vi "Puzzle 16-2 right.vi"() -> ()   [LabVIEW 2022 SP3]
panel:
  in  "delimited string":string="\\.........-......|...../................................-...........|.../.\\\\...\\|...................|.........\n../..\\...............-../............\\.........-......-................././........|......................|...\n......../..-........../................../...|.....-......................\\.....-..............|............/|\n......-......-............................\\..\\............../................./.-.................\\.....|.\\|..\n...-....-|....................-...-..../...................-....../...........|.............\\.....-...........\n..\\............../..../................|...........|/......|..........-\\.........|...../....................|.\n\\...........\\.\\....../...|..........--.................|......//...../..-.....|.....-.........................\n..................................................|...........\\.\\.................../.....................\\...\n.....-...................-............./.......................|............/...|..........................-..\n..............-......\\..............\\................................-.|../................|....|../\\....|....\n./../\\..............-..............|.........................|\\................................|.-./.....|....\n..........\\....-................./........../............../........\\-..........\\....-........................\n.........-....../.............\\../-......-.............\\........\\......./......-|..\\.........\\............-...\n......-....|.......|.............................\\..-.............\\......-......................|......|......\n....\\......../.............................||....-.............-.........................\\........../.........\n........-......................................................\\.........../...|./............-|..............\n......\\..-........|./..................\\../....|.........-\\...-..-....\\...-................\\..................\n|./.....\\.-......../.-|.............\\..\\.\\......-.|............/.|..\\|....................../.................\n................................../..-........\\.\\..|.-..|/...-...............-............\\........-..../.....\n.......|............\\../......\\...../.......................|........|...-.|...\\...-....\\......|..............\n.................-......./........../.......|/........|....-\\........../..............-................../....\n..../...................-..\\.........|................../..|.../...............|-\\............../.............\n.............................|....../............................|..|.........../....../....-.|..||....\\......\n.....//.........\\..........\\.|...-./.......|.-..\\...\\.......\\.-.............../.....|..............-.|........\n.-...........\\.\\..........\\|..\\.....\\.|...........--.............\\.....-./.......\\................../.........\n............\\....................................\\.......-....../.....\\....../....-.....................-.....\n\\.......\\...-.|......./\\..|...\\......|......../.....-.....|......./................./.........../.............\n/.|.....................................................\\./.........\\...|......|.......................|./..-.\n....|............./....\\...-.\\...../.......\\.................|.............|......\\..../.../..\\...........\\...\n..........................|...........|.../............\\..\\....\\............-|...................\\.../......\\.\n.......|\\.\\............./...../.......././..../.....-..|...\\.......|..........\\............/-.................\n.|\\....|.....-.-......\\-..........\\.....................\\...........................-...|.....|..-...........|\n/\\......|....-.............................-/....|..|........./.........................................../.-.\n...............................|....................||....|.|....|./............./.|........./............\\...\n.......-......................./.............\\....-....-...-..\\........................................-......\n.......-....|.........../................-.....................................|............../...............\n.-..................\\.../...../\\...\\.......................\\...............-...//..\\......\\-.|..........|.....\n..\\............................././\\............../....-..........|..\\....\\.-./...............................\n...-.|/...........||......\\...-.........................................|.....................................\n......|.././...........|......................./.||................\\........\\........|.|.....\\...|....|.......\n...-......./............../.....|..-..-.|..-.......|..|....................\\...\\.......\\........|.............\n/../.................|............................/.............../....-/..|.....\\...|........................\n.........-.........|............/.......-.............-...../.\\|.......\\...-..\\.-.....|..../...........-\\..|..\n......................................\\........|..../....|.......\\......-.................|...................\n...\\.......|.....|....\\....................-............-....|......\\.........\\...................|...........\n.....\\.............\\...-........|.............................-|......./.........-............//.......|......\n............/../...........-/.........................-...|...|...\\............./....-..|..........\\\\.........\n..\\......................\\/./.........................\\..-............-\\..-...................................\n............................\\...|.........|...|.\\.......|............/.........|.................\\............\n............|..|...........\\..................../........|............-....-./.....\\.-..-.................../.\n...................-.-.......-.\\............-....\\........-./.|../|.../.............\\.......\\............-....\n..../............../........../\\...............-.............../......|.\\/.........../......|.................\n...\\......\\.....................\\..|...............-.......................-.-|....../..................-.....\n.........\\...\\.............|........../.........................................................-...\\......-..\n..-...........-\\.........\\....\\.............../........\\./........../....\\......../...........................\n............|.............-.../.................|......../..-.........../............./...................\\..\\\n........-...................................-.....\\-.........|............../..../...\\\\.|..........\\....-.....\n..\\..\\.\\.\\.........../..|...\\............/...|......................-.........................|...............\n\\.../...../..........|.....\\...|./...|............./......\\........................-.....-.....\\..............\n|....................-..-............................../...../..............-.../...-...|../../.\\.............\n................/......-...|....|..........\\\\......-..............|\\........|./.\\...|.......................|.\n........../....................|./..........................|..................-.........|.........|..........\n..../.....\\...|.......|../....................\\...\\..-...\\...\\...........|............./.-.....--.............\n.........|-..........................\\..-......--......../................\\......\\...../.|...|....../....-....\n.......|.............\\............./...............././/../..........\\.........|\\..........|..................\n....\\........|.../......./....\\./...//.............\\..................|./.....................................\n..........-.|\\............/..-...........\\........-....|....../........-.|.................-/.-.........|.../|\n.....-\\........\\........|.|...............................-...........\\./..........................-........\\.\n............../........./../--|.........................-....................\\......-..\\...\\..........\\......\\\n..|...............................\\........\\......\\..\\.....-\\............|....................................\n..\\|.................\\-......|...............\\.........|.|...|........................|..../......-...-|...-..\n...........................\\......................-.............................|........./......./....-......\n.........-..../........../.......|../.....-.........................../.../...........|....-./.\\..............\n.-........./..-/...........\\.......-.......-.........//.-.-......................................|...-........\n........../.....|...........\\....../\\............-......-......../....................|......................-\n.......||....-.../....|....../....-.......|...................................................................\n.....|./........\\.-.....|..................|....\\....../......\\.......-|.....|../....\\...\\.\\........|./......-\n.-.|./............-....../............-..................|....|......-.....\\................||.\\\\.............\n....-...-........./.........../.........\\....|.\\....|..\\.\\............................-.......//......\\..-.\\..\n...../.........................................|..........|.-|..\\./............\\.-.../......./............-..|\n.../..........\\..............\\..../...\\.........\\................./.|....../........|............-...-.-..../.\n..\\.\\................\\....../....................|......../\\|...../...\\....-..../...\\.....|..../...\\..........\n......\\..-.\\........................-.....................-............|.|.............-...-..................\n................\\...\\...../../....../.../................/.........\\.\\.................|......................\n......................|..................-./.........\\..\\.......-..........|..\\.......\\...-...|...............\n..........-.........................-................................./......../.....-.|......................\n.......-\\............./...............-............|.....................-..\\.................-......\\....-...\n..........................................\\......./......\\........-|..|.....\\........\\......./................\n........//...........-........../......./..............|...../..-..................../...\\......-..........-..\n./....|..-|...|......-.............\\.|.........................\\...............-\\.............................\n|....................|....................../............................../...........\\...|...-..............\n\\......./....|.../.|....................|..............|..................|................\\..................\n.........|......\\.............../....\\...................................|.\\........./..-.................|./.\n......../..................\\..................../.........................||./.-.............../..............\n......................./.........|.|........-../........./.....|............./......|......-....|...../.......\n................|......./............\\...-......../..................\\..\\..../.......\\.../.........-/.........\n.........-.....\\......-.....................-..-.........//...........................|...\\-............../...\n.....|............-...../.\\......................|........|...........\\..........|./......./.\\.........\\../...\n..\\..........-.../.......|......./.................../............\\............|......../....|................\n.....\\....................-...........-......//...........\\....|..\\...-.....................\\.............../.\n..-.....|......\\.......|.../......................\\...|...\\..\\.....|...........................\\..........|...\n....-....-...|.\\-...-..\\............../......-./...........\\/............\\-..|.........................\\......\n......./.....-|.|.......|....\\|||......\\.............................................\\......-.................\n.................-\\................/.-...............|............|...|.-......-..............................\n...|.............|...............|.......-.................-.........|.../..................................|.\n..-.../.....-.........................-....|......|/...../....\\.............................-...............-.\n.|.........-../....................../............|................\\.....|........\\...........................\n.\\\\............\\................-../.../....\\.................................|.-.....|.....\\.........-.....|.\n.............../..................../..\\.............-..\\.......\\...\\..../..-........-..../-.....|............\n\\.................................-..............|...\\./......../...........................|.........|......."
  out "Array 3":i32[](array[numeric])
  out "max value":i32
  out "size":i32
  in  "Array 2":cluster{"Array 3":string[]}[](array[cluster])=[{"Array 3"=["v"]}, {"Array 3"=["^"]}, {"Array 3"=["^", "v"]}, {"Array 3"=["<"]}, {"Array 3"=["<"]}, {"Array 3"=["^"]}, {"Array 3"=["v"]}, {"Array 3"=["^", "v"]}, {"Array 3"=[">"]}, {"Array 3"=[">"]}, {"Array 3"=[">"]}, {"Array 3"=["<"]}, {"Array 3"=["^"]}, {"Array 3"=["<", ">"]}, {"Array 3"=["^"]}, {"Array 3"=["<"]}, {"Array 3"=[">"]}, {"Array 3"=["v"]}, {"Array 3"=["<", ">"]}, {"Array 3"=["v"]}]
  out "Array":T1(array[cluster])
  out "character array":string[][](array[string])
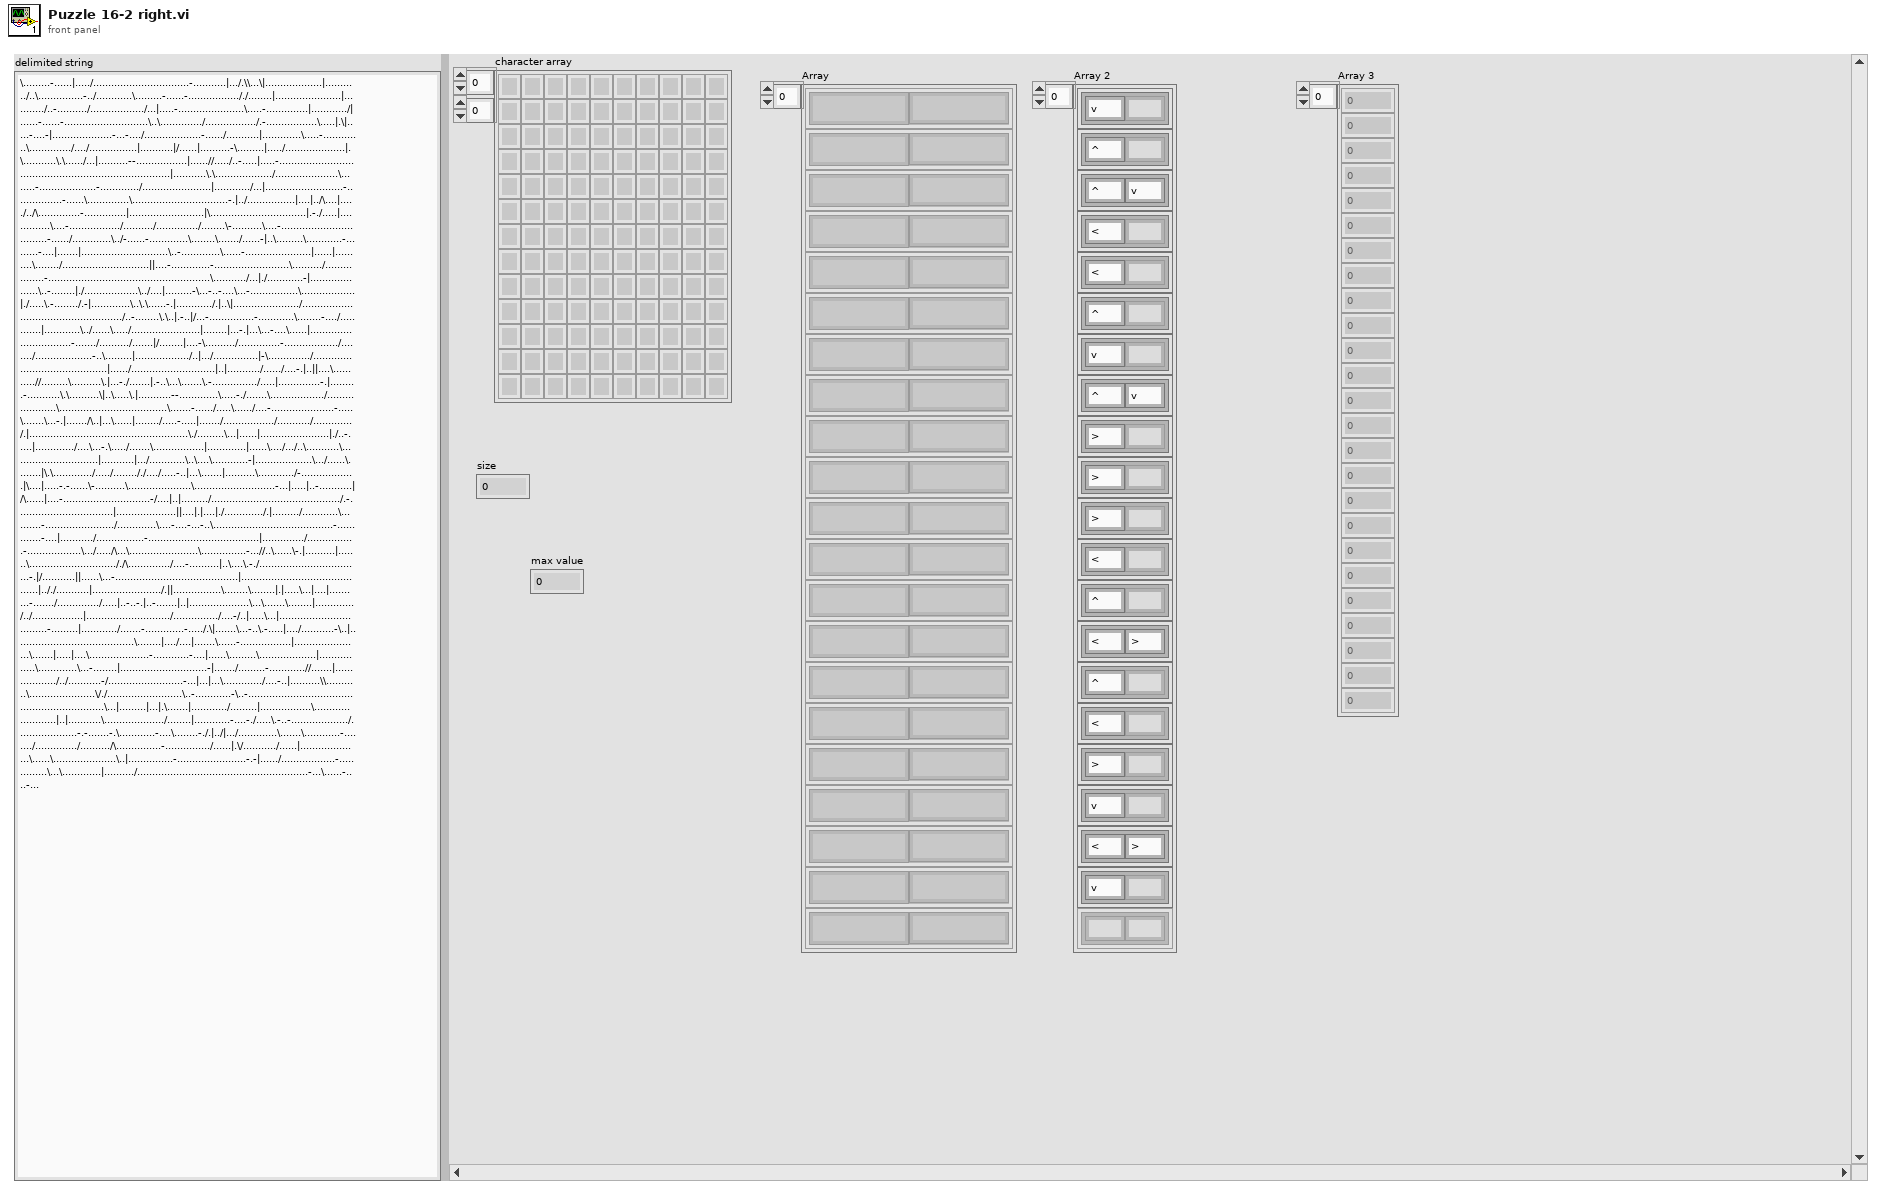
[diagram p1: front panel]
types:
  T1 = cluster{"input string":string, "input string":string}[]
  T2 = map{cluster{"input string":string, "input string 2":string}, string[]}
  T3 = cluster{"input string":string, "input string":string}
  T4 = set{cluster{cluster{i32, i32}, "input string":string}}
  T5 = cluster{cluster{i32, i32}, "input string":string}
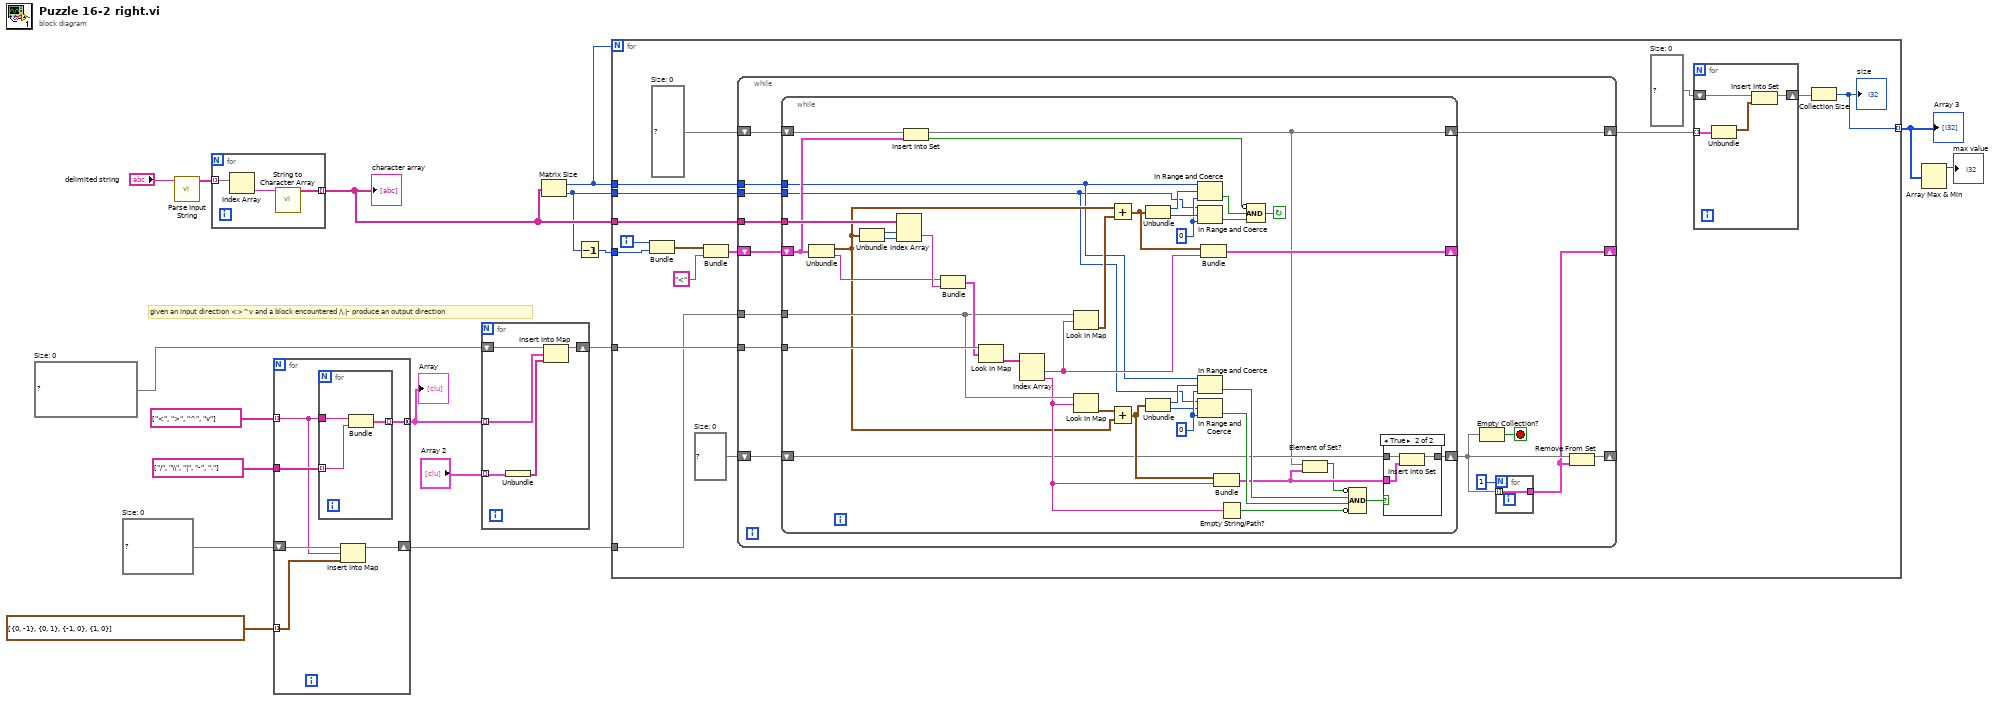
[diagram p0: block diagram]
diagram:
  w9 = map{string, cluster{i32, i32}} {}  # Size: 0
  w11 = T2 {}  # Size: 0
  # "given an input direction <>^v and a block encountered /\\.|- produce an output direction"
  n1 = call "Parse Input String.vi"("delimited string"="delimited string") -> ("parsed string"=w16:string[][])  [unwired: 10 in]
  n2 = for {
    tunnel: w16 -> [w20] mode=indexing
    tunnel: [w18] -> w6 mode=indexing
    n3 = Index Array(array=w20) -> (element=w19:string)  [unwired: 1 in]
    n4 = call "String to Character Array.vi"("input string"=w19) -> ("character array"=w18:string[])  [unwired: 10 in]
  }
  "character array" <- w6
  n5 = for {
    tunnel: string[] ["<", ">", "^", "v"] ("character array") -> [w22] mode=indexing
    tunnel: string[] ["/", "\\", "|", "-", "."] ("character array") -> [w26]
    tunnel: [w25] -> w13 mode=concatenating
    tunnel: cluster{i32, i32}[] [{0, -1}, {0, 1}, {-1, 0}, {1, 0}] -> [w21] mode=indexing
    shift-right: [w23] -> w7
    shift-left: w9 -> [w24]
    n6 = for {
      tunnel: w22 -> [w29]
      tunnel: w26 -> [w28] mode=indexing
      tunnel: [w27] -> w25 mode=indexing
      n7 = Bundle("input string"=w29, "input string"=w28) -> (w27:T3)  [unwired: 1 in]
    }
    n8 = Insert Into Map(map in=w24, key=w22, value=w21) -> (map out=w23:map{string, cluster{i32, i32}})  [unwired: 2 out]
  }
  "Array" <- w13
  n9 = for {
    tunnel: w13 -> [w32] mode=indexing
    tunnel: "Array 2" -> [w31] mode=indexing
    shift-right: [w33] -> w8
    shift-left: w11 -> [w34]
    n10 = Unbundle(w31) -> ("Array 3"=w30:string[])
    n11 = Insert Into Map(map in=w34, key=w32, value=w30) -> (map out=w33:T2)  [unwired: 2 out]
  }
  n12 = Matrix Size(0:w6) -> (1:w5:i32, 2:w2:i32)
  n13 = Decrement(x=w2) -> (x-1=w1:i32)
  n14 = for {
    N: w5 -> [_]
    tunnel: w8 -> [w49]
    tunnel: w7 -> [w48]
    tunnel: w6 -> [w47]
    tunnel: w5 -> [w46]
    tunnel: w2 -> [w45]
    tunnel: [w36] -> w4 mode=indexing
    tunnel: w1 -> [w35]
    i -> [w38]
    w39 = T4 {}  # Size: 0
    w41 = set{cluster{i32, i32}} {}  # Size: 0
    w50 = T4 {}  # Size: 0
    n15 = Bundle(w38, w35) -> (w37:cluster{i32, i32})  [unwired: 1 in]
    n16 = Bundle(w37, "input string"="<") -> (w43:T5)  [unwired: 1 in]
    n17 = while {
      tunnel: w49 -> [w66]
      tunnel: w48 -> [w65]
      tunnel: w47 -> [w64]
      shift-right: [w63] -> w42
      shift-left: w50 -> [w67]
      shift-right: [w55] -> _
      shift-left: w43 -> [w68]
      shift-right: [w56] -> _
      shift-left: w39 -> [w60]
      tunnel: w46 -> [w62]
      tunnel: w45 -> [w61]
      stop <- w59 stop-if-true
      n18 = while {
        shift-right: [w91] -> _
        shift-left: w68 -> [w94]
        shift-right: [w72] -> w63
        shift-left: w67 -> [w109]
        tunnel: w64 -> [w108]
        tunnel: w66 -> [w104]
        tunnel: w65 -> [w88]
        tunnel: w62 -> [w81]
        tunnel: w61 -> [w80]
        shift-right: [w73] -> w57
        shift-left: w60 -> [w74]
        stop <- w100 continue-if-true
        w84 = 0 ("lower limit")
        w96 = 0 ("lower limit")
        n19 = Unbundle(w94) -> (w85:cluster{i32, i32}, "input string"=w95:string)
        n20 = Unbundle(w85) -> (w107:i32, w106:i32)
        n21 = Index Array(array=w108, index (row)=w107, index (col)=w106) -> (element=w105:string)
        n22 = Insert Into Set(10:w94, 11:w109) -> (2:w90:bool, 3:w72:T4)
        n23 = Bundle("input string"=w95, "input string"=w105) -> (w103:T3)  [unwired: 1 in]
        n24 = Look In Map(map=w104, key=w103) -> (value=w102:string[])  [unwired: 1 in, 1 out]
        n25 = Index Array(array=w102) -> (element #1=w93:string, element #2=w87:string)  [unwired: 2 in]
        n26 = Look In Map(map=w88, key=w93) -> (value=w89:cluster{i32, i32})  [unwired: 1 in, 1 out]
        n27 = Look In Map(map=w88, key=w87) -> (value=w86:cluster{i32, i32})  [unwired: 1 in, 1 out]
        n28 = Add(x=w85, y=w89) -> (x+y=w92:cluster{i32, i32})
        n29 = Add(x=w86, y=w85) -> (x+y=w79:cluster{i32, i32})
        n30 = Unbundle(w92) -> (w99:i32, w101:i32)
        n31 = Unbundle(w79) -> (w83:i32, w82:i32)
        n32 = In Range and Coerce(upper limit=w81, x=w99, lower limit=w96) -> (In Range?=w98:bool)  [unwired: 1 out]
        n33 = In Range and Coerce(upper limit=w80, x=w101, lower limit=w96) -> (In Range?=w97:bool)  [unwired: 1 out]
        n34 = In Range and Coerce(upper limit=w81, x=w83, lower limit=w84) -> (In Range?=w76:bool)  [unwired: 1 out]
        n35 = In Range and Coerce(upper limit=w80, x=w82, lower limit=w84) -> (In Range?=w77:bool)  [unwired: 1 out]
        n36 = Bundle(w92, "input string"=w93) -> (w91:T5)  [unwired: 1 in]
        n37 = Bundle(w79, "input string"=w87) -> (w71:T5)  [unwired: 1 in]
        n38 = Empty String/Path?(string/path=w87) -> (empty?=w78:bool)
        n39 = Compound Arithmetic op=AND(invert w90, w98, w97) -> (w100:bool)
        n40 = Element of Set?(10:w71, 11:w72) -> (3:w70:bool)
        n41 = Compound Arithmetic op=AND(invert w70, w76, w77, invert w78) -> (w75:bool)
        n42 = case shown="True" w75 {
          tunnel: w71 -> [_ w112]
          tunnel: w74 -> [w110 w113]
          tunnel: [w110 w111] -> w73
          frame False {
          }
          frame True {
            n43 = Insert Into Set(10:w112, 11:w113) -> (3:w111:T4)  [unwired: 1 out]
          }
        }
      }
      n44 = Empty Collection?(1:w57) -> (0:w59:bool)
      n45 = for {
        N: 1 -> [_]
        tunnel: w57 -> [w69] mode=indexing
        tunnel: [w69] -> w55
      }
      n46 = Remove From Set(10:w55, 11:w57) -> (3:w56:T4)  [unwired: 1 out]
    }
    n47 = for {
      tunnel: w42 -> [w54] mode=indexing
      shift-right: [w51] -> w40
      shift-left: w41 -> [w53]
      n48 = Unbundle(w54) -> (w52:cluster{i32, i32})  [unwired: 1 out]
      n49 = Insert Into Set(10:w52, 11:w53) -> (3:w51:set{cluster{i32, i32}})  [unwired: 1 out]
    }
    n50 = Collection Size(1:w40) -> (0:w36:i32)
    "size" <- w36
  }
  "Array 3" <- w4
  n51 = Array Max & Min(array=w4) -> (max value=→"max value":i32)  [unwired: 3 out]
